vi "CRYChange Plot Property.vi"(6 "Items":u16, 7 "sOption":string, 8 "Control Ref":refnum<vi>, 9 "pProperty VI":refnum<vi>, 10 "pGraph VI In":refnum<vi>, 11 "ControlName In":string) -> (3 "ControlName Out":string)   [LabVIEW 2013]
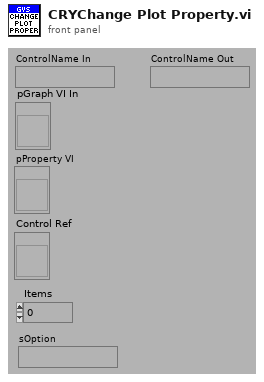
[diagram p1: front panel]
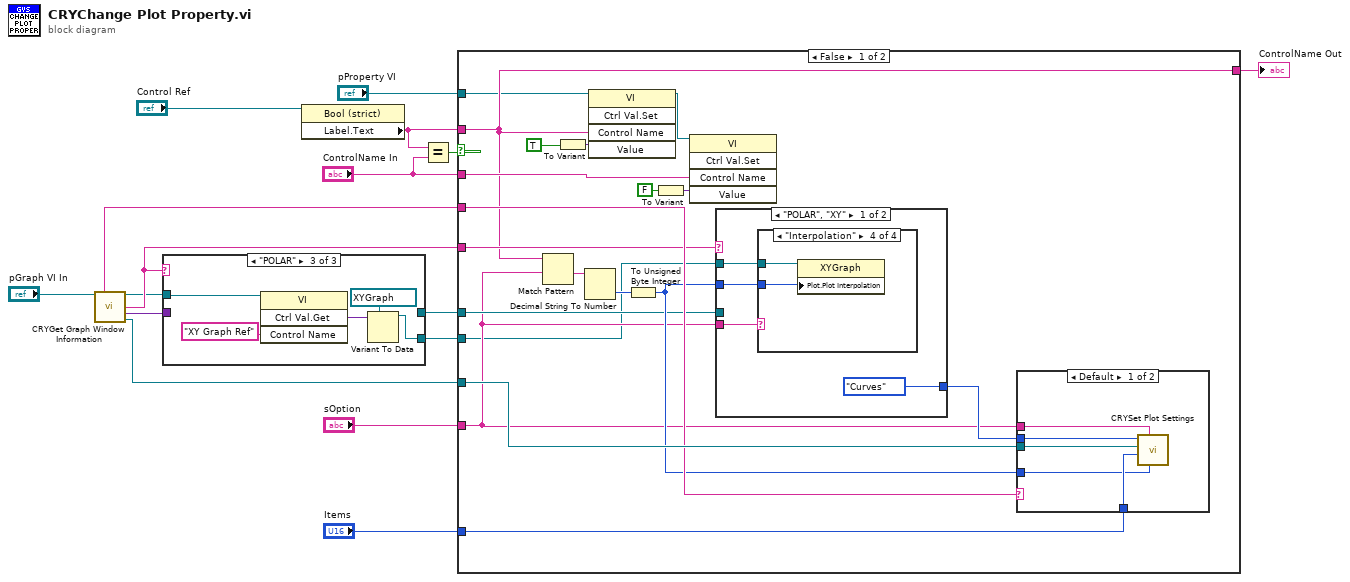
[diagram p0: block diagram]
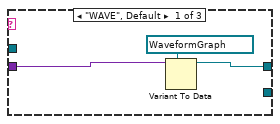
[diagram p2: hidden frame]
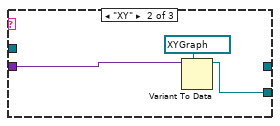
[diagram p3: hidden frame]
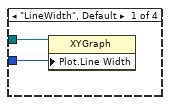
[diagram p4: hidden frame]
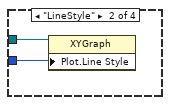
[diagram p5: hidden frame]
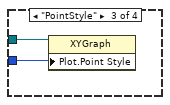
[diagram p6: hidden frame]
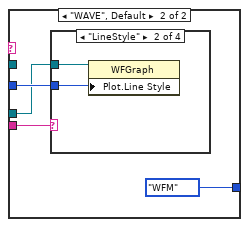
[diagram p7: hidden frame]
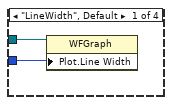
[diagram p8: hidden frame]
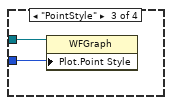
[diagram p9: hidden frame]
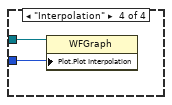
[diagram p10: hidden frame]
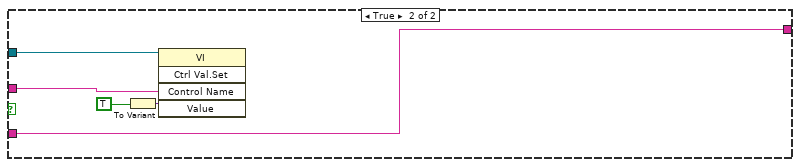
[diagram p12: hidden frame]
diagram:
  n1 = call "CRYGet Graph Window Information.vi"("pGraph VI In"="pGraph VI In") -> ("Queue Name Out"=w11:string, "pGraph VI Out"=w1:refnum<vi>, "Graph Type Out"=w8:string, "Graph Control Ref Out"=w9:variant, "Legend Ref Out"=w10:refnum<vi>)  [unwired: 4 in, 6 out]
  n2 = case shown="\"POLAR\"" w8 {
    tunnel: w9 -> [w19 w22 _]
    tunnel: [w17 _ _] -> w5
    tunnel: [_ w20 w26] -> w7
    tunnel: w1 -> [_ _ w23]
    frame "WAVE", Default {
      n3 = Variant To Data(type=refnum<vi> refnum ("Legend Ref"), Variant=w19) -> (data=w17:refnum<vi>)  [unwired: 1 in, 1 out]
    }
    frame "XY" {
      n4 = Variant To Data(type=refnum<vi> refnum ("Legend Ref"), Variant=w22) -> (data=w20:refnum<vi>)  [unwired: 1 in, 1 out]
    }
    frame "POLAR" {
      n5 = invoke class="VI" method="Ctrl Val.Get"(reference=w23, "Control Name"="XY Graph Ref") -> ("Get Control Value Variant"=w24:variant)  [unwired: 2 in, 3 out]
      n6 = Variant To Data(type=refnum<vi> refnum ("Legend Ref"), Variant=w24) -> (data=w26:refnum<vi>)  [unwired: 1 in, 1 out]
    }
  }
  n7 = property class="Bool (strict)"(reference="Control Ref") -> ("Label.Text"=w15:string)  [unwired: 1 in, 2 out]
  n8 = Equal?(x=w15, y="ControlName In") -> (x = y?=w16:bool)
  n9 = case shown="False" w16 {
    tunnel: w15 -> [w33 w78]
    tunnel: "ControlName In" -> [w46 w76]
    tunnel: w10 -> [w38 _]
    tunnel: w11 -> [w37 _]
    tunnel: "Items" -> [w35 _]
    tunnel: w7 -> [w28 _]
    tunnel: "pProperty VI" -> [w30 w77]
    tunnel: w8 -> [w34 _]
    tunnel: [w33 w76] -> w6
    tunnel: w5 -> [w31 _]
    tunnel: "sOption" -> [w29 _]
    frame False {
      n10 = Match Pattern(string=w33, regular expression=w29) -> (after substring=w39:string)  [unwired: 4 out]
      n11 = To Variant(anything=TRUE) -> (Variant=w44:variant)
      n12 = Decimal String To Number(string=w39) -> (number=w40:i32)  [unwired: 3 out]
      n13 = invoke class="VI" method="Ctrl Val.Set"(reference=w30, "Control Name"=w33, "Value"=w44) -> (reference out=w45:refnum<vi>)  [unwired: 2 in, 4 out]
      n14 = To Unsigned Byte Integer(number=w40) -> (unsigned 8bit integer=w36:u8)
      n15 = To Variant(anything=FALSE) -> (Variant=w42:variant)
      n16 = invoke class="VI" method="Ctrl Val.Set"(reference=w45, "Control Name"=w46, "Value"=w42) -> ()  [unwired: 2 in, 5 out]
      n17 = case shown="\"POLAR\", \"XY\"" w34 {
        tunnel: w36 -> [w50 w62]
        tunnel: w28 -> [w49 _]
        tunnel: [enum16{"Curves", "Values", "Results", "WFM"}."Curves" ("Type") enum16{"Curves", "Values", "Results", "WFM"}."WFM" ("Type")] -> w32
        tunnel: w31 -> [_ w59]
        tunnel: w29 -> [w47 w60]
        frame "POLAR", "XY" {
          n18 = case shown="\"Interpolation\"" w47 {
            tunnel: w50 -> [w52 w54 w56 w58]
            tunnel: w49 -> [w51 w53 w55 w57]
            frame "LineWidth", Default {
              n19 = property class="XYGraph"(reference=w51, "Plot.Line Width"=w52) -> ()  [unwired: 1 in, 2 out]
            }
            frame "LineStyle" {
              n20 = property class="XYGraph"(reference=w53, "Plot.Line Style"=w54) -> ()  [unwired: 1 in, 2 out]
            }
            frame "PointStyle" {
              n21 = property class="XYGraph"(reference=w55, "Plot.Point Style"=w56) -> ()  [unwired: 1 in, 2 out]
            }
            frame "Interpolation" {
              n22 = property class="XYGraph"(reference=w57, "Plot.Plot Interpolation"=w58) -> ()  [unwired: 1 in, 2 out]
            }
          }
        }
        frame "WAVE", Default {
          n23 = case shown="\"LineStyle\"" w60 {
            tunnel: w62 -> [w64 w66 w68 w70]
            tunnel: w59 -> [w63 w65 w67 w69]
            frame "LineWidth", Default {
              n24 = property class="WFGraph"(reference=w63, "Plot.Line Width"=w64) -> ()  [unwired: 1 in, 2 out]
            }
            frame "LineStyle" {
              n25 = property class="WFGraph"(reference=w65, "Plot.Line Style"=w66) -> ()  [unwired: 1 in, 2 out]
            }
            frame "PointStyle" {
              n26 = property class="WFGraph"(reference=w67, "Plot.Point Style"=w68) -> ()  [unwired: 1 in, 2 out]
            }
            frame "Interpolation" {
              n27 = property class="WFGraph"(reference=w69, "Plot.Plot Interpolation"=w70) -> ()  [unwired: 1 in, 2 out]
            }
          }
        }
      }
      n28 = case shown="Default" w37 {
        tunnel: w38 -> [w75 _]
        tunnel: w36 -> [w73 _]
        tunnel: w35 -> [w74 _]
        tunnel: w32 -> [w72 _]
        tunnel: w29 -> [w71 _]
        frame Default {
          n29 = call "CRYSet Plot Settings.vi"("Style"=w73, "sAction"=w71, "Row"=w74, "Legend Refnum"=w75, "Type"=w72) -> ()  [unwired: 2 in, 5 out]
        }
        frame "ViewReport" {
        }
      }
    }
    frame True {
      n30 = To Variant(anything=TRUE) -> (Variant=w80:variant)
      n31 = invoke class="VI" method="Ctrl Val.Set"(reference=w77, "Control Name"=w78, "Value"=w80) -> ()  [unwired: 2 in, 5 out]
    }
  }
  "ControlName Out" <- w6
